vi "Needle Valve labVIEW Code-Original.vi"() -> ()   [LabVIEW 2025]
uses:
  e7797c04-791b-4eea-89a1-5a3bec2431d3.vi
  bf5fd3a0-ddf8-478e-bb95-a39885d33854.vi
  0285ecf2-4d18-4427-ace1-61b1951a0741.vi
  843b8d60-a9e3-46f8-8afe-ca8ffa5d81a2.vi
  fe75afdf-d463-4dd5-8739-de0ca1ff0544.vi
  <vilib>/gmath/NI_Gmath.lvlib
  d3b0afdc-d7ac-4f1a-8ecc-0aeb21fe1e80.vi
  c8945bc9-af31-4a2e-9b52-27840c61c0f1.vi
  <vilib>/Utility/file.llb/Write Delimited Spreadsheet (DBL).vi
  <vilib>/Utility/file.llb/Read Delimited Spreadsheet (DBL).vi
  <vilib>/addons/_office/excel.llb/Excel Easy Table (num).vi
  <vilib>/Utility/NIReport.llb/NI_report.lvclass
  <vilib>/Utility/NIReport.llb/Report Type.ctl
  <vilib>/Utility/NIReport.llb/NI_ReportGenerationCore.lvlib
  0d300616-a92e-4ad7-b5ed-aabe3c94486a.vi
  <vilib>/Instr/_visa.llb/VISA Configure Serial Port (Instr).vi
  <vilib>/addons/_office/excel.llb/Excel Easy Table (str).vi
panel:
  in  "Sensor Values Excel Sheet Name":string
  in  "?":u32(colorbox)
  out "Waveform Chart":dbl[](graph)
  in  "Loop Iteration":i32
  in  "Saved Sensor Values":path
  in  "Mach 2.1 Table Excel Sheet Name":string
  in  "Mach 3.0 Table Excel Sheet Name":string
  out "Mach # duration (s)":dbl
  in  "Mach Tables Location":path
  out "Output Mach #\n(For Reference Only)":dbl format="%#_4g"
  out "Motor Signal":string
  out "?":dbl format="%.4f"
  out "Output Mach #\n(For Reference Only)":dbl format="%#_4g"
  out "Motor Signal":string
  out "?":dbl format="%.3f"
  in  "Seclect Spike":enum16{"Mach 2.1 Spike", "Mach 3.0 Spike"}(ring)
  in  "?":dbl
  out "Motor Signal":string
  in  "?":dbl[][](array[numeric])=[[10.0, 10.0, 0.0, 22.0]]
  in  "stop program":bool
  in  "?":bool
  out "?":dbl format="%.4f"
  in  "Select Mach Number":dbl[](array[numeric])
  out "Spike Position":dbl[][](graph)
  out "Arduino Error":errorcluster
  in  "VISA resource Port":refnum<visa-resource-name>
  out "?":dbl format="%.3f"
  out "?":dbl format="%.3f"
  in  "Set Spike Position (in)":dbl(slide) scale=0.0..0.5
  in  "Mach Number, Spike Distance (in) (3.0M)":dbl[][](array[numeric])=[[10.0, 10.0, 0.0, 22.0]]
  in  "Mach Number, Spike Distance (in) (2.1M)":dbl[][](array[numeric])=[[10.0, 10.0, 0.0, 22.0]]
  out "?":dbl(slide) scale=0.0..1000.0
  out "Stagnation Flow Temp (K)\n(For Refrence only)":dbl
  out "Stagnation pressure (PSIA)\n(For Refrence only)":dbl
  in  "Sensor Offsets":dbl[](array[numeric])=[10.0, 10.0, 0.0, 22.0]
  in  "Sensor K-values":dbl[](array[numeric])=[10.0, 10.0, 0.0, 22.0]
  in  "?":bool
  in  "?":bool
  in  "?":bool
  out "Screw RPM (95% efficency assumed)":dbl
  out "Spike Linear Speed (in/s)\n(For Reference Only)":dbl format="%#_4g"
  in  "Motor Control Loop Rate (ms)":dbl
  out "Set Motor RPM":dbl(knob) scale=0.0..200.0
  in  "Flight Profile Mode":bool
  in  "Set Mach # Mode":bool
  in  "Manual Positioning Mode":bool
  in  "Stop Sensors":bool
  in  "Sensor Loop Rate (ms)":dbl
  out "Time Since Start (s)\n(For Reference Only)":dbl format="%.2f"
  in  "loop stop 2":bool
  in  "loop stop 1":bool
  in  "Sensor Inputs Location":path
  in  "Start Sensors":bool
  in  "Load Inputs":bool
  in  "Save Inputs":bool
  out "Potentiometer distance\n(For Reference Only)":dbl
  out "Port":i32
  out "ConnectionType":i32
  out "DeviceType":i32
  out "Labjack error":errorcluster
  # "34HS59-6004S Motor Torque Curve (For Reference)"
  # "Labjack/Arduino Resources"
  # "Inputs and LabJack Sensor Monitors"
  # "Mach Number Tables"
  # "Mach 3.0 Spike Table"
  # "Mach 2.1 Spike Table"
  # "Motor RPM >200 RPM"
  # "Potentiometer"
  # "Inefficent Torque for High Mass Flow/Thrust Tests"
  # "Ducer"
  # "Thermocouple"
  # "Motor RPM < 200 RPM"
  # "(Labjack Auto-Populates)"
  # "(dial indicator for range reference)"
  # "COM Port for Arduino"
  # "Stop sensors automatically saves sensor data"
  # "Distance to Go (in)\n(For Reference Only)"
  # "Output Mach #\n(For Reference Only)"
  # "Column one: selected Mach numbers"
  # "Profile Control Array"
  # "Column Two: selected timing for each Mach number (seconds)"
  # "Distance to Go (in)\n(For Reference Only)"
  # "Profile will be completed at first Mach number = \"0\""
  # "Distance to Go (in)\n(For Reference Only)"
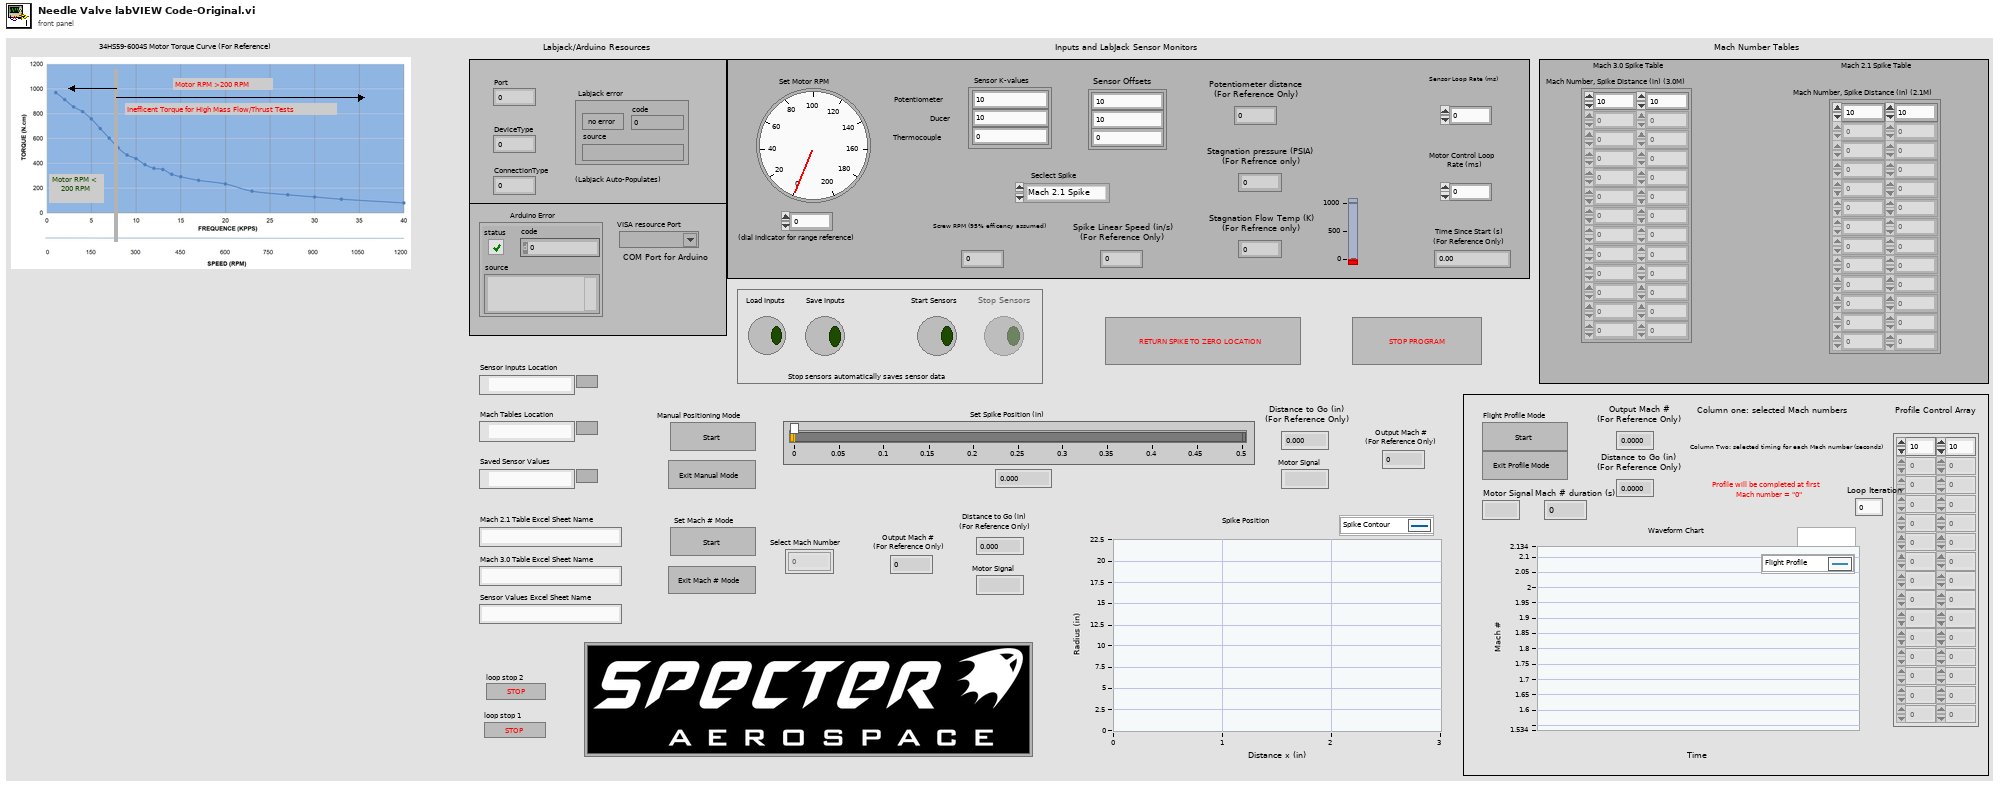
[diagram p1: front panel]
types:
  T1 = enum16{"Save Data", "Idle Mode", "Manual Positioning Mode", "Set Mach # mode", "Flight Profile Mode"}
  T2 = enum16{"save data", "Start sensors", "save values", "load Values", "Idle"}
  T3 = enum8{"Enabled", "Disabled", "Disabled and Grayed Out"}
  T4 = typedef "NI_ReportGenerationCore.lvlib/Report Type.ctl" = enum16{"HTML", "Word", "Excel"}
  T5 = enum16{"Left Button", "Center Button", "Right Button", "Window Close"}
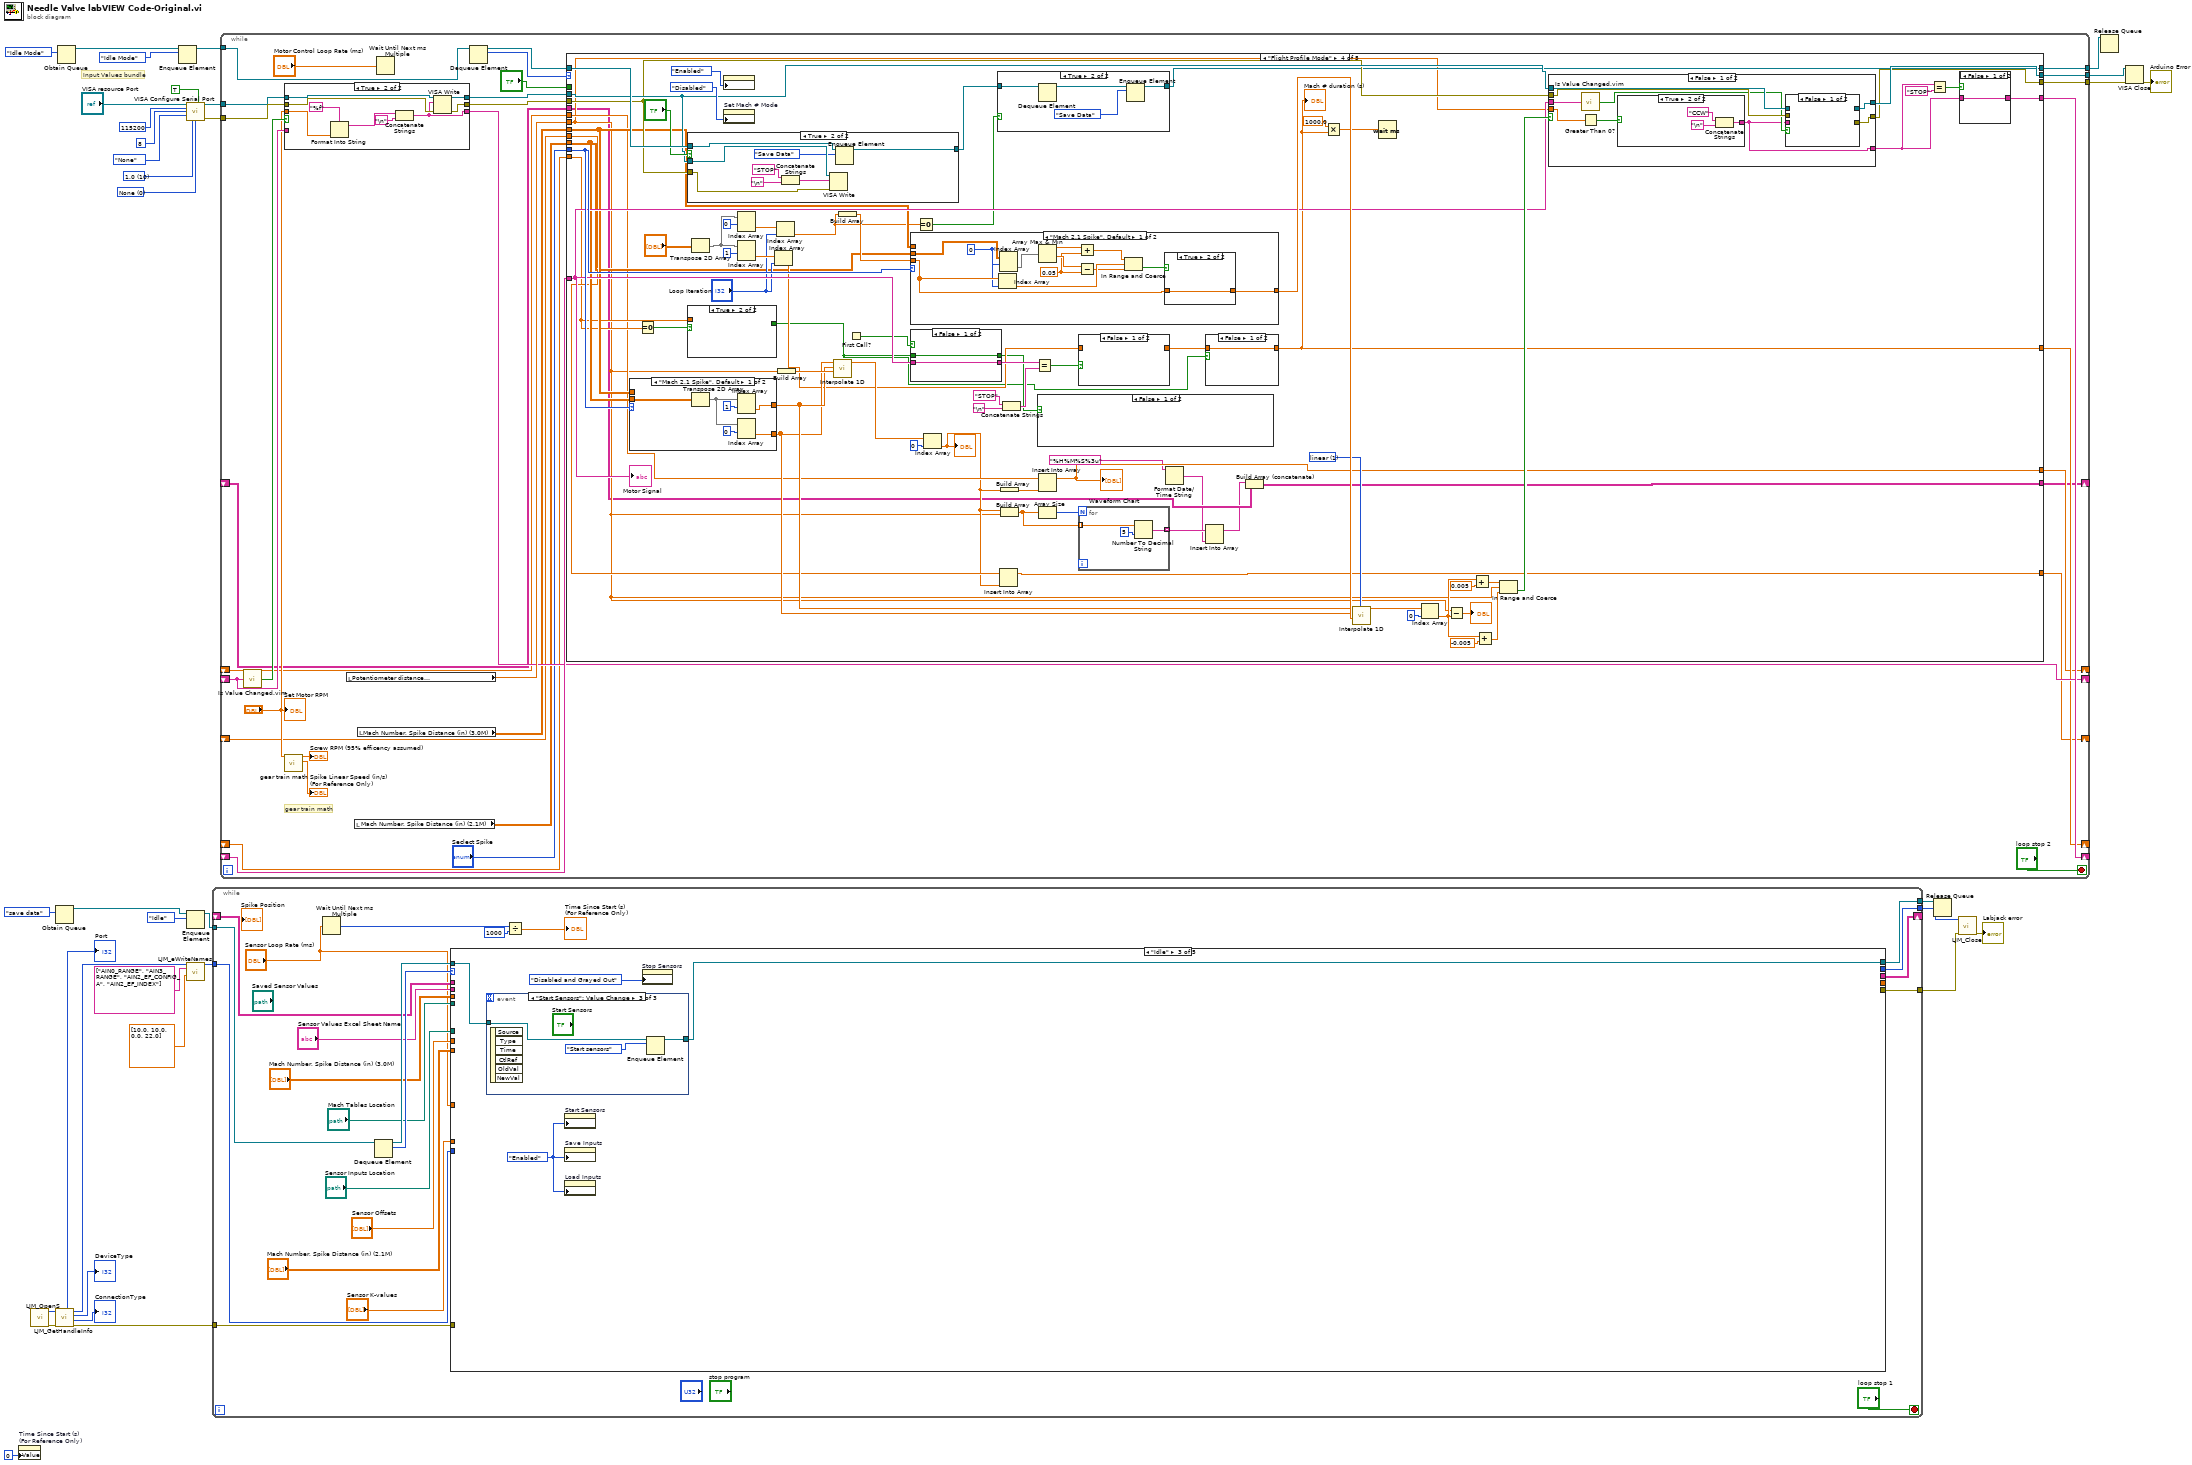
[diagram p0: block diagram]
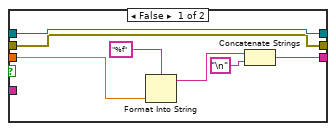
[diagram p2: hidden frame]
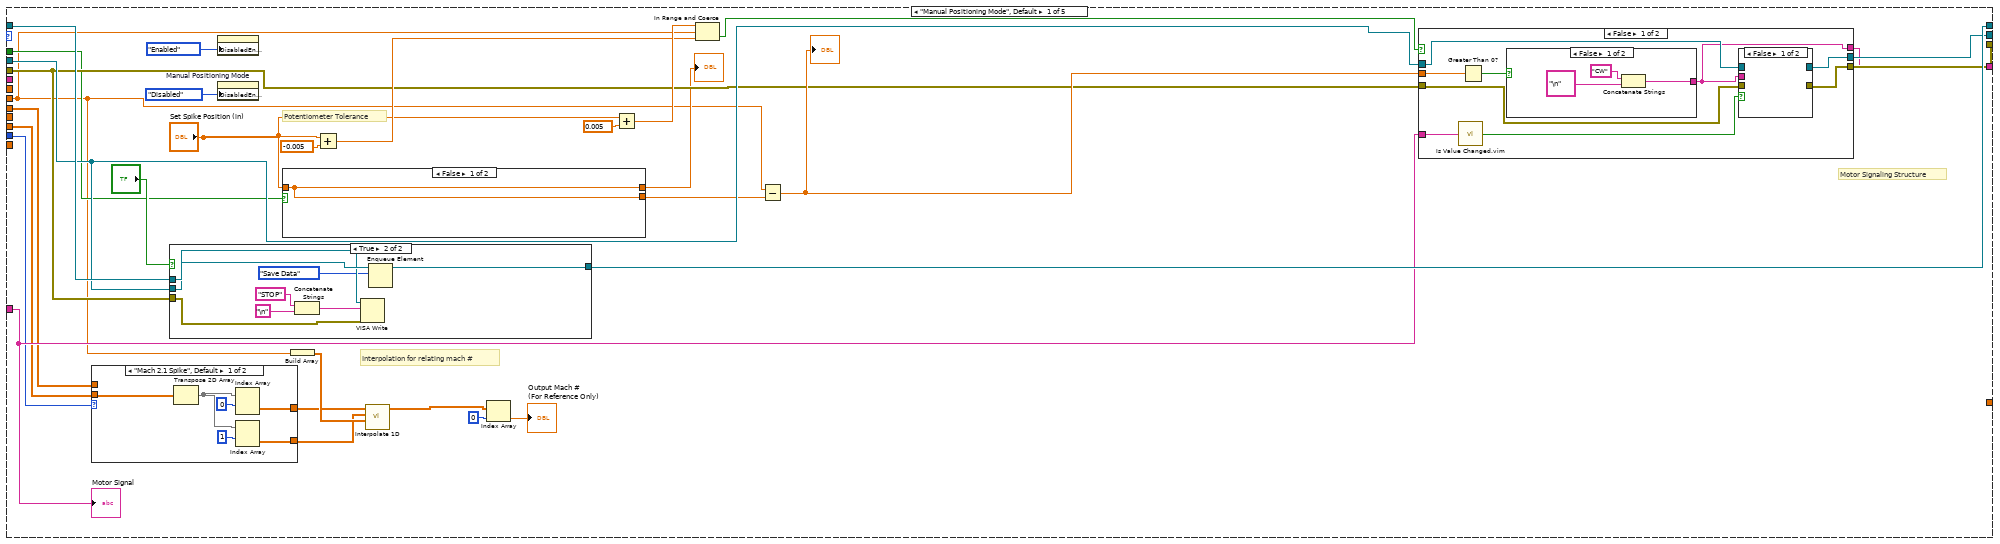
[diagram p3: hidden frame]
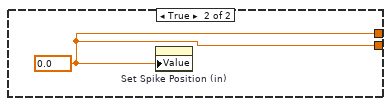
[diagram p4: hidden frame]
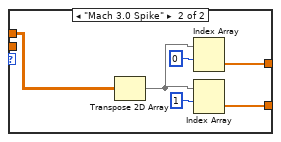
[diagram p5: hidden frame]
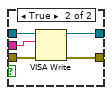
[diagram p6: hidden frame]
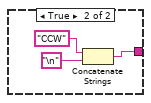
[diagram p7: hidden frame]
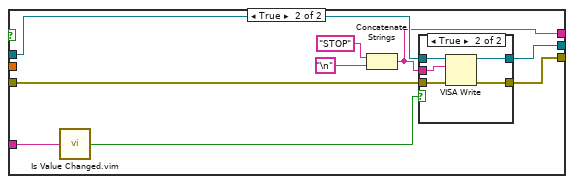
[diagram p8: hidden frame]
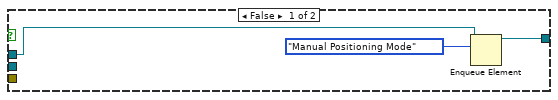
[diagram p10: hidden frame]
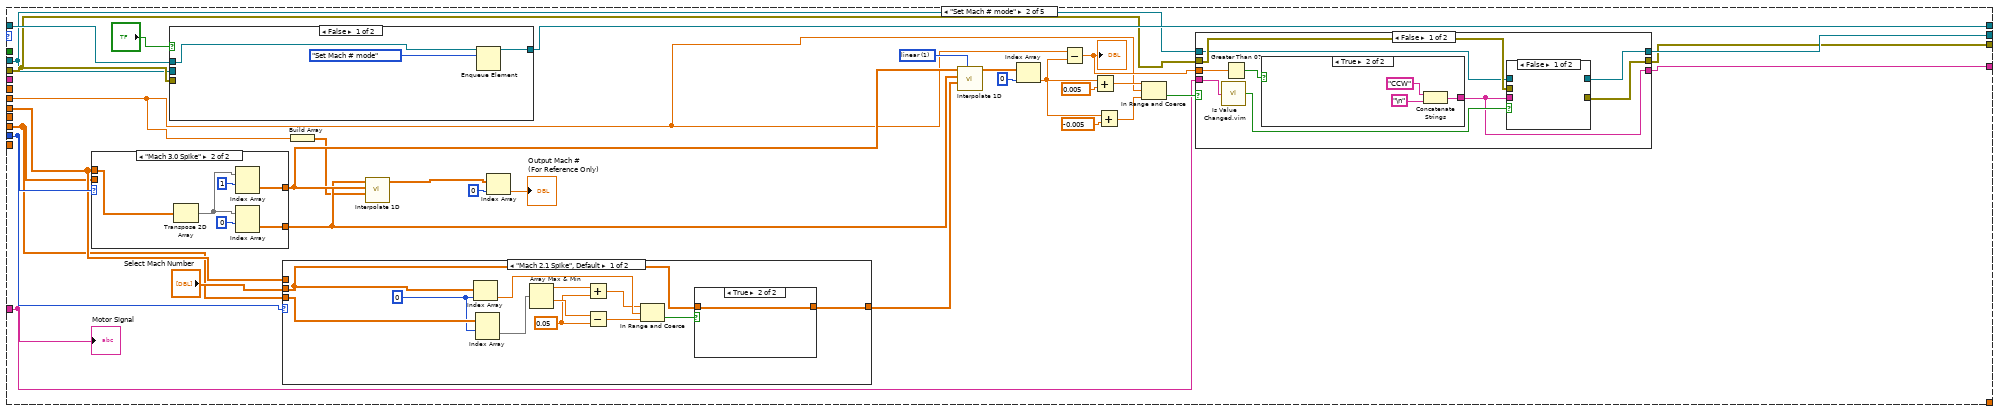
[diagram p11: hidden frame]
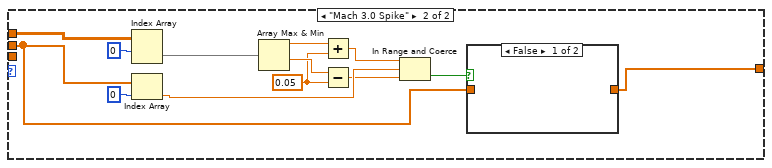
[diagram p13: hidden frame]
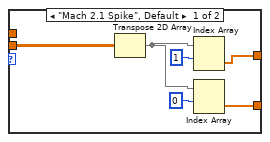
[diagram p15: hidden frame]
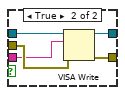
[diagram p16: hidden frame]
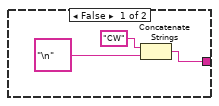
[diagram p17: hidden frame]
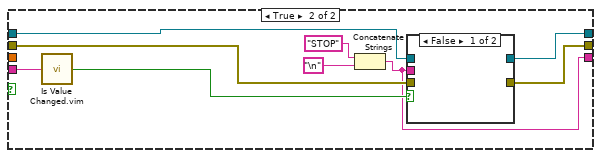
[diagram p18: hidden frame]
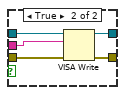
[diagram p19: hidden frame]
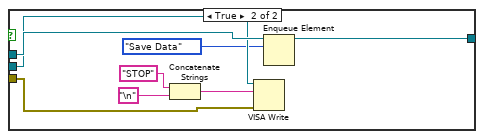
[diagram p20: hidden frame]
diagram:
  w5 = u16 0 items=["None", "XON/XOFF", "RTS/CTS", "XON/XOFF & RTS/CTS", "DTR/DSR", "XON/XOFF & DTR/DSR"] ("flow control (0:none)")
  w6 = u16 10 items=["1.0"=10, "1.5"=15, "2.0"=20] ("stop bits (10: 1 bit)")
  # "Input Values bundle"
  n1 = property on="Time Since Start (s)\n(For Reference Only)" class="DigNum (strict)"("Value"=u32 0 ("Time Since Start (s)\n(For Reference Only) 2")) -> ()  [unwired: 2 in, 2 out]
  n2 = call "LJM_OpenS.vi"() -> ("error out"=w31:errorcluster, "Handle"=w35:i32)  [unwired: 10 in]
  n3 = Obtain Queue(element data type=T2."save data" ("Enum")) -> (queue out=w24:refnum<queue>)  [unwired: 4 in, 2 out]
  n4 = call "LJM_GetHandleInfo.vi"("error in"=w31, "Handle In"=w35) -> ("error out"=w30:errorcluster, "ConnectionType"=→"ConnectionType":i32, "DeviceType"=→"DeviceType":i32, "Handle Out"=w17:i32, "Port"=→"Port":i32)  [unwired: 2 in, 3 out]
  n5 = Obtain Queue(element data type=T1."Idle Mode") -> (queue out=w26:refnum<queue>)  [unwired: 4 in, 2 out]
  n6 = Enqueue Element(queue=w26, element=T1."Idle Mode") -> (queue out=w25:refnum<queue>)  [unwired: 2 in, 2 out]
  n7 = call-poly "VISA Configure Serial Port"("VISA resource name"="VISA resource Port", "Enable Termination\nChar (T)"=TRUE ("Enable Termination\nChar (T)"), "baud rate (9600)"=u32 115200, "data bits (8)"=u16 8, "parity (0:none)"=enum16{"None", "Odd", "Even", "Mark", "Space"}."None", "stop bits (10: 1 bit)"=w6, "flow control (0:none)"=w5) -> ("VISA resource name out"=w3:refnum<visa-resource-name>, "error out"=w4:errorcluster)  [unwired: 7 in]
  n8 = Enqueue Element(queue=w24, element=T2."Idle" ("Enum")) -> (queue out=w23:refnum<queue>)  [unwired: 2 in, 2 out]
  n9 = call "LJM_eWriteNames.vi"("Handle In"=w17, "aNames"=string[] ["AIN0_RANGE", "AIN3_RANGE", "AIN2_EF_CONFIG_A", "AIN2_EF_INDEX"], "aValuesIn"=dbl[] [10.0, 10.0, 0.0, 22.0]) -> ("Handle Out"=w16:i32)  [unwired: 10 in, 2 out]
  n10 = while {
    tunnel: w30 -> [w58]
    tunnel: [w57] -> w29
    tunnel: w16 -> [w56]
    tunnel: [w55] -> w28
    tunnel: w23 -> [w54]
    tunnel: [w51] -> w21
    shift-right: [w40] -> _
    shift-left: _ -> [w39]
    stop <- "loop stop 1" stop-if-true
    n11 = Wait Until Next ms Multiple(millisecond multiple="Sensor Loop Rate (ms)") -> (millisecond timer value=w49:u32)
    n12 = Dequeue Element(queue=w54) -> (queue out=w52:refnum<queue>, element=w53:T2)  [unwired: 2 in, 2 out]
    n13 = case shown="\"Idle\"" w53 {
      tunnel: w58 -> [_ _ _ w180 _]
      tunnel: [_ _ _ w179 _] -> w57
      tunnel: w56 -> [_ _ _ w182 _]
      tunnel: [_ _ _ w181 _] -> w55
      tunnel: w52 -> [w80 w115 w150 w187 w211]
      tunnel: [w79 w114 w149 w186 w209] -> w51
      tunnel: [_ _ _ w171 _] -> _
      tunnel: "Sensor Offsets" -> [w76 _ _ w176 _]
      tunnel: "Sensor K-values" -> [w75 _ _ w175 _]
      tunnel: "Sensor Inputs Location" -> [w72 w112 _ _ _]
      tunnel: "Mach Tables Location" -> [w69 w111 _ _ _]
      tunnel: "Mach Number, Spike Distance (in) (2.1M)" -> [w68 _ _ _ _]
      tunnel: "Mach Number, Spike Distance (in) (3.0M)" -> [w70 _ _ _ _]
      tunnel: [_ _ _ w163 _] -> w40
      tunnel: w39 -> [_ _ _ w162 w204]
      tunnel: "Sensor Values Excel Sheet Name" -> [_ _ _ _ w202]
      tunnel: "Sensor Loop Rate (ms)" -> [w60 _ _ _ _]
      frame "save values", Default {
        w63 = string[] ["Mach #", "Spike Distance (in)"] ("column headers")
        w74 = Report_Type."Excel" ("report type")
        n14 = local read "Motor Control Loop Rate (ms)"() -> (w62:dbl)
        n15 = Enqueue Element(queue=w80, element=T2."Idle" ("Enum")) -> (queue out=w79:refnum<queue>)  [unwired: 2 in, 2 out]
        n16 = local read "Set Motor RPM"() -> (w73:dbl)
        n17 = Build Array(w60) -> (w59:dbl[])
        n18 = Build Array(w62) -> (w61:dbl[])
        n19 = Build Array(w73) -> (w77:dbl[])
        n20 = Build Array(w75, w76, w77, w59, w61) -> (w71:dbl[][])
        n21 = flat-sequence {
          tunnel: w72 -> [w84]
          tunnel: w71 -> [w83]
          tunnel: w69 -> [w93]
          tunnel: w70 -> [w92]
          tunnel: w65 -> [w89]
          tunnel: "Mach 3.0 Table Excel Sheet Name" -> [w88]
          tunnel: w63 -> [w87]
          tunnel: w69 -> [w105]
          tunnel: w68 -> [w104]
          tunnel: w67 -> [w101]
          tunnel: "Mach 2.1 Table Excel Sheet Name" -> [w100]
          tunnel: w63 -> [w99]
          frame #0 {
            n22 = Two Button Dialog(message="Save Sensor Values/Inputs?" ("Message")) -> (T button?=w82:bool)  [unwired: 2 in]
            n23 = case shown="True" w82 {
              tunnel: w84 -> [_ w86]
              tunnel: w83 -> [_ w85]
              frame False {
              }
              frame True {
                n24 = call-poly <vilib>:"Write Delimited Spreadsheet.vi"("file path (dialog if empty)"=w86, "2D data"=w85) -> ()  [unwired: 12 in, 2 out]
              }
            }
          }
          frame #1 {
            n25 = Two Button Dialog(message="Save Mach 3.0 Table" ("Message")) -> (T button?=w90:bool)  [unwired: 2 in]
            n26 = case shown="True" w90 {
              tunnel: w93 -> [_ w98]
              tunnel: w92 -> [_ w96]
              tunnel: w89 -> [_ w97]
              tunnel: w88 -> [_ w95]
              tunnel: w87 -> [_ w94]
              frame False {
              }
              frame True {
                n27 = call-poly <vilib>:"Write Delimited Spreadsheet.vi"("file path (dialog if empty)"=w98, "2D data"=w96) -> ()  [unwired: 12 in, 2 out]
                n28 = call-poly <vilib>:"Excel Easy Table.vi"("report in"=w97, "text data"=w96, "name (\"\")"=w95, "column headers"=w94) -> ()  [unwired: 7 in, 5 out]
              }
            }
          }
          frame #2 {
            n29 = Two Button Dialog(message="Save Mach 2.1 Table" ("Message")) -> (T button?=w102:bool)  [unwired: 2 in]
            n30 = case shown="True" w102 {
              tunnel: w105 -> [_ w110]
              tunnel: w104 -> [_ w108]
              tunnel: w101 -> [_ w109]
              tunnel: w100 -> [_ w107]
              tunnel: w99 -> [_ w106]
              frame False {
              }
              frame True {
                n31 = call-poly <vilib>:"Excel Easy Table.vi"("report in"=w109, "text data"=w108, "name (\"\")"=w107, "column headers"=w106) -> ()  [unwired: 7 in, 5 out]
                n32 = call-poly <vilib>:"Write Delimited Spreadsheet.vi"("file path (dialog if empty)"=w110, "2D data"=w108) -> ()  [unwired: 12 in, 2 out]
              }
            }
          }
        }
        n33 = call <vilib>:"Create Report.vi"("Report Type"=w74) -> ("report out"=w65:refnum<class "NI_report.lvclass">)  [unwired: 13 in, 1 out]
        n34 = call <vilib>:"Create Report.vi"("Report Type"=w74) -> ("report out"=w67:refnum<class "NI_report.lvclass">)  [unwired: 13 in, 1 out]
      }
      frame "load Values" {
        n35 = flat-sequence {
          tunnel: w112 -> [w118]
          tunnel: w111 -> [w139]
          tunnel: w111 -> [w144]
          frame #0 {
            n36 = Two Button Dialog(message="Sensor and RPM File Selection" ("Message")) -> (T button?=w116:bool)  [unwired: 2 in]
            n37 = case shown="True" w116 {
              tunnel: w118 -> [_ w128]
              frame False {
              }
              frame True {
                # "Loading Motor RPM"
                n38 = call-poly <vilib>:"Read Delimited Spreadsheet.vi"("file path (dialog if empty)"=w128) -> ("all rows"=w120:dbl[][])  [unwired: 9 in, 5 out]
                n39 = Index Array(array=w120, index (row)=0) -> (element=w135:dbl[])  [unwired: 1 in]
                n40 = Index Array(array=w120, index (row)=2) -> (element=w131:dbl[])  [unwired: 1 in]
                n41 = Index Array(array=w120, index (row)=1) -> (element=w133:dbl[])  [unwired: 1 in]
                n42 = property on="Sensor K-values" class="Arr (strict)"("Value"=w135) -> ()  [unwired: 2 in, 2 out]
                n43 = property on="Sensor Offsets" class="Arr (strict)"("Value"=w133) -> ()  [unwired: 2 in, 2 out]
                n44 = Index Array(array=w120, index (row)=3) -> (element=w126:dbl[])  [unwired: 1 in]
                n45 = Index Array(array=w120, index (row)=4) -> (element=w122:dbl[])  [unwired: 1 in]
                n46 = Index Array(array=w131, index=0) -> (element=w129:dbl)
                n47 = property class="DigNum (strict)"("Value"=w129) -> ()  [unwired: 2 in, 2 out]
                n48 = Index Array(array=w126, index=0) -> (element=w124:dbl)
                n49 = Index Array(array=w122, index=0) -> (element=w119:dbl)
                n50 = property on="Motor Control Loop Rate (ms)" class="DigNum (strict)"("Value"=w119) -> ()  [unwired: 2 in, 2 out]
                n51 = property on="Sensor Loop Rate (ms)" class="DigNum (strict)"("Value"=w124) -> ()  [unwired: 2 in, 2 out]
              }
            }
          }
          frame #1 {
            n52 = Two Button Dialog(message="Mach 2.1 Table Selection" ("Message")) -> (T button?=w137:bool)  [unwired: 2 in]
            n53 = case shown="True" w137 {
              tunnel: w139 -> [_ w140]
              frame False {
              }
              frame True {
                n54 = call-poly <vilib>:"Read Delimited Spreadsheet.vi"("file path (dialog if empty)"=w140) -> ("all rows"=w141:dbl[][])  [unwired: 9 in, 5 out]
                n55 = property on="Mach Number, Spike Distance (in) (2.1M)" class="Arr (strict)"("Value"=w141) -> ()  [unwired: 2 in, 2 out]
              }
            }
          }
          frame #2 {
            n56 = Two Button Dialog(message="Mach 3.0 Table Selection" ("Message")) -> (T button?=w142:bool)  [unwired: 2 in]
            n57 = case shown="True" w142 {
              tunnel: w144 -> [_ w146]
              frame False {
              }
              frame True {
                n58 = call-poly <vilib>:"Read Delimited Spreadsheet.vi"("file path (dialog if empty)"=w146) -> ("all rows"=w145:dbl[][])  [unwired: 9 in, 5 out]
                n59 = property on="Mach Number, Spike Distance (in) (3.0M)" class="Arr (strict)"("Value"=w145) -> ()  [unwired: 2 in, 2 out]
              }
            }
          }
        }
        n60 = Enqueue Element(queue=w115, element=T2."Idle" ("Enum")) -> (queue out=w114:refnum<queue>)  [unwired: 2 in, 2 out]
      }
      frame "Idle" {
        w148 = T3."Enabled" ("Disabled")
        n61 = event shown="[2] \"Start Sensors\": Value Change" {
          selector: _ -> [_ _ _]
          dyn-events: _ -> [_ _ _]
          timeout: _ -> [_ _ _]
          tunnel: w150 -> [w153 w156 w159]
          tunnel: [w152 w155 w158] -> w149
          event "Save Inputs": Value Change {
            n62 = event-data() -> ()  [unwired: 1 in, 6 out]
            n63 = Enqueue Element(queue=w153, element=T2."save values" ("Enum")) -> (queue out=w152:refnum<queue>)  [unwired: 2 in, 2 out]
          }
          event "Load Inputs": Value Change {
            n64 = event-data() -> ()  [unwired: 1 in, 6 out]
            n65 = Enqueue Element(queue=w156, element=T2."load Values" ("Enum")) -> (queue out=w155:refnum<queue>)  [unwired: 2 in, 2 out]
          }
          event "Start Sensors": Value Change {
            n66 = event-data() -> ()  [unwired: 1 in, 6 out]
            n67 = Enqueue Element(queue=w159, element=T2."Start sensors" ("Enum")) -> (queue out=w158:refnum<queue>)  [unwired: 2 in, 2 out]
          }
        }
        n68 = property on="Start Sensors" class="Bool"("DisabledEnum"=w148) -> ()  [unwired: 2 in, 2 out]
        n69 = property on="Save Inputs" class="Bool"("DisabledEnum"=w148) -> ()  [unwired: 2 in, 2 out]
        n70 = property on="Load Inputs" class="Bool"("DisabledEnum"=w148) -> ()  [unwired: 2 in, 2 out]
        n71 = property on="Stop Sensors" class="Bool"("DisabledEnum"=T3."Disabled and Grayed Out" ("Disabled")) -> ()  [unwired: 2 in, 2 out]
      }
      frame "Start sensors" {
        (unwired) 5 ("sample length")
        w184 = T3."Disabled and Grayed Out" ("Disabled")
        # "Sensor Calibration and LabJack Read"
        n72 = Array Size(array=w176) -> (size(s)=w177:i32)
        n73 = property on="Stop Sensors" class="Bool"("DisabledEnum"=T3."Enabled" ("Disabled")) -> ()  [unwired: 2 in, 2 out]
        n74 = call "LJM_eReadNames.vi"("Handle In"=w182, "aNames"=string[] ["AIN0", "AIN3", "AIN2_EF_READ_A"], "error in"=w180) -> ("Handle Out"=w181:i32, "aValuesOut"=w168:dbl[], "error out"=w179:errorcluster)  [unwired: 9 in, 1 out]
        n75 = property on="Save Inputs" class="Bool"("DisabledEnum"=w184) -> ()  [unwired: 2 in, 2 out]
        n76 = property on="Start Sensors" class="Bool"("DisabledEnum"=w184) -> ()  [unwired: 2 in, 2 out]
        n77 = property on="Load Inputs" class="Bool"("DisabledEnum"=w184) -> ()  [unwired: 2 in, 2 out]
        n78 = for {
          N: w177 -> [_]
          tunnel: w176 -> [w192] mode=indexing
          tunnel: w175 -> [w193] mode=indexing
          tunnel: w168 -> [w195] mode=indexing
          tunnel: [w191] -> w166 mode=indexing
          n79 = Multiply(x=w193, y=w195) -> (x*y=w194:dbl)
          n80 = Add(x=w192, y=w194) -> (x+y=w191:dbl)
        }
        n81 = case shown="True" "Stop Sensors" {
          tunnel: w187 -> [w198 w201]
          tunnel: [w197 w200] -> w186
          frame False {
            n82 = Enqueue Element(queue=w198, element=T2."Start sensors" ("Enum")) -> (queue out=w197:refnum<queue>)  [unwired: 2 in, 2 out]
          }
          frame True {
            n83 = Enqueue Element(queue=w201, element=T2."save data") -> (queue out=w200:refnum<queue>)  [unwired: 2 in, 2 out]
          }
        }
        n84 = Array Size(array=w166) -> (size(s)=w167:i32)
        n85 = Index Array(array=w166, index=enum16{"Potentiometer", "Ducer", "Thermocouple"}."Potentiometer" ("Enum")) -> (element=w171:dbl)
        "Potentiometer distance\n(For Reference Only)" <- w171
        n86 = Index Array(array=w166, index=enum16{"Potentiometer", "Ducer", "Thermocouple"}."Thermocouple" ("Enum")) -> (element=→"?" →"Stagnation Flow Temp (K)\n(For Refrence only)":dbl)
        n87 = for {
          N: w167 -> [_]
          tunnel: w166 -> [w190] mode=indexing
          tunnel: [w188] -> w165 mode=indexing
          n88 = Number To Decimal String(number=w190, width (-)=i16 5) -> (decimal integer string=w188:string)
        }
        n89 = Index Array(array=w166, index=enum16{"Potentiometer", "Ducer", "Thermocouple"}."Ducer" ("Enum")) -> (element=→"Stagnation pressure (PSIA)\n(For Refrence only)":dbl)
        n90 = Format Date/Time String(time format string (%c)="%H%M%S%3u") -> (date/time string=w160:string)  [unwired: 2 in]
        n91 = Insert Into Array(array=w165, new element=w160) -> (w164:string[])  [unwired: 1 in]
        n92 = Build Array (concatenate)(w164, w162) -> (w163:string[][])
      }
      frame "save data" {
        n93 = Enqueue Element(queue=w211, element=T2."Idle") -> (queue out=w209:refnum<queue>)  [unwired: 2 in, 2 out]
        n94 = Two Button Dialog(message="Save sensor Values?" ("Message")) -> (T button?=w207:bool)  [unwired: 2 in]
        n95 = call <vilib>:"Create Report.vi"("Report Type"=Report_Type."Excel" ("report type")) -> ("report out"=w206:refnum<class "NI_report.lvclass">)  [unwired: 13 in, 1 out]
        n96 = case shown="True" w207 {
          tunnel: w206 -> [_ w213]
          tunnel: string[] ["Spike position (in)", "Flow Pressure (PSIA)", "Flow Temperature (K)", "Time (s)"] ("column headers") -> [_ w215]
          tunnel: w204 -> [_ w214]
          tunnel: w202 -> [_ w212]
          frame False {
          }
          frame True {
            n97 = call-poly <vilib>:"Excel Easy Table.vi"("report in"=w213, "text data"=w214, "name (\"\")"=w212, "column headers"=w215) -> ()  [unwired: 7 in, 5 out]
          }
        }
      }
    }
    n98 = Divide(x=w49, y=u32 1000) -> (x/y=→"Time Since Start (s)\n(For Reference Only)":dbl)
  }
  n99 = while {
    tunnel: w25 -> [w248]
    tunnel: [w246] -> w20
    tunnel: [w241] -> w11
    tunnel: [w240] -> w10
    shift-right: [w239] -> _
    shift-left: _ -> [w238]
    tunnel: w4 -> [w237]
    tunnel: w3 -> [w236]
    shift-right: [w232] -> _
    shift-left: _ -> [w231]
    shift-right: [w223] -> _
    shift-left: _ -> [w222]
    shift-right: [w221] -> _
    shift-left: _ -> [w220]
    shift-right: [w219] -> _
    shift-left: _ -> [w218]
    shift-right: [w217] -> _
    shift-left: _ -> [w216]
    stop <- "loop stop 2" stop-if-true
    # "gear train math"
    n100 = call "Is Value Changed.vim"("value"=w231) -> ("changed or first call?"=w233:bool)
    n101 = case shown="True" w233 {
      tunnel: w237 -> [w254 w264]
      tunnel: [w250 w256] -> w232
      tunnel: w236 -> [w255 w263]
      tunnel: [w254 w262] -> w235
      tunnel: [w255 w259] -> w234
      tunnel: "?" -> [w253 w261]
      tunnel: w231 -> [_ _]
      frame False {
        n102 = Format Into String(format string="%f", w253) -> (resulting string=w251:string)  [unwired: 2 in, 1 out]
        n103 = Concatenate Strings(w251, "\n" ("string")) -> (w250:string)
      }
      frame True {
        n104 = Format Into String(format string="%f", w261) -> (resulting string=w258:string)  [unwired: 2 in, 1 out]
        n105 = Concatenate Strings(w258, "\n" ("string")) -> (w256:string)
        n106 = VISA Write(VISA resource name=w263, write buffer=w256, error in (no error)=w264) -> (VISA resource name out=w259:refnum<visa-resource-name>, error out=w262:errorcluster)  [unwired: 1 out]
      }
    }
    n107 = call "gear train math.vi"("Numeric in"="?") -> ("Numeric 3"=→"Spike Linear Speed (in/s)\n(For Reference Only)":dbl, "Numeric out"=→"Screw RPM (95% efficency assumed)":dbl)  [unwired: 9 in]
    n108 = local read "Potentiometer distance\n(For Reference Only)"() -> (w242:dbl)
    n109 = local read "Mach Number, Spike Distance (in) (2.1M)"() -> (w225:dbl[][])
    n110 = local read "Mach Number, Spike Distance (in) (3.0M)"() -> (w224:dbl[][])
    n111 = Wait Until Next ms Multiple(millisecond multiple="Motor Control Loop Rate (ms)") -> ()  [unwired: 1 out]
    n112 = Dequeue Element(queue=w248) -> (queue out=w245:refnum<queue>, element=w247:T1)  [unwired: 2 in, 2 out]
    n113 = case shown="\"Flight Profile Mode\"" w247 {
      tunnel: [w294 w379 w480 w514 w677] -> w246
      tunnel: w245 -> [w295 w378 w481 w564 w679]
      tunnel: w242 -> [w265 w358 _ w499 _]
      tunnel: w234 -> [w282 w376 w472 w546 _]
      tunnel: [w286 w375 w472 w549 _] -> w241
      tunnel: w235 -> [w281 w377 w471 w545 _]
      tunnel: [w285 w374 w471 w548 _] -> w240
      tunnel: [w284 w373 _ w542 _] -> w239
      tunnel: w238 -> [w283 w372 _ w538 _]
      tunnel: "Seclect Spike" -> [w278 w369 _ w550 _]
      tunnel: w225 -> [w277 w355 _ w517 _]
      tunnel: w224 -> [w276 w356 _ w518 _]
      tunnel: "?" -> [w269 _ _ _ _]
      tunnel: [_ _ _ w510 _] -> w223
      tunnel: w222 -> [_ _ _ w505 _]
      tunnel: [_ _ _ w506 _] -> w221
      tunnel: w220 -> [_ _ _ w507 _]
      tunnel: [_ _ _ w502 _] -> w219
      tunnel: w218 -> [_ _ _ w501 _]
      tunnel: [_ _ _ w497 _] -> w217
      tunnel: w216 -> [_ _ _ w496 w673]
      frame "Manual Positioning Mode", Default {
        # "Motor Signaling Structure"
        # "Potentiometer Tolerance"
        # "Interpolation for relating mach #"
        n114 = case shown="\"Mach 2.1 Spike\", Default" w278 {
          tunnel: w277 -> [w301 _]
          tunnel: [w303 w308] -> w274
          tunnel: [w302 w309] -> w273
          tunnel: w276 -> [_ w305]
          frame "Mach 2.1 Spike", Default {
            n115 = Transpose 2D Array(2D array=w301) -> (transposed array=w300:dbl[][])
            n116 = Index Array(array=w300, index (row)=0) -> (element=w302:dbl[])  [unwired: 1 in]
            n117 = Index Array(array=w300, index (row)=1) -> (element=w303:dbl[])  [unwired: 1 in]
          }
          frame "Mach 3.0 Spike" {
            n118 = Transpose 2D Array(2D array=w305) -> (transposed array=w304:dbl[][])
            n119 = Index Array(array=w304, index (row)=0) -> (element=w309:dbl[])  [unwired: 1 in]
            n120 = Index Array(array=w304, index (row)=1) -> (element=w308:dbl[])  [unwired: 1 in]
          }
        }
        n121 = case shown="True" "?" {
          tunnel: w295 -> [w346 w354]
          tunnel: [w345 w353] -> w294
          tunnel: w282 -> [_ w349]
          tunnel: w281 -> [_ w348]
          frame False {
            n122 = Enqueue Element(queue=w346, element=T1."Manual Positioning Mode") -> (queue out=w345:refnum<queue>)  [unwired: 2 in, 2 out]
          }
          frame True {
            n123 = Concatenate Strings("STOP" ("write buffer"), "\n" ("write buffer")) -> (w352:string)
            n124 = VISA Write(VISA resource name=w349, write buffer=w352, error in (no error)=w348) -> ()  [unwired: 3 out]
            n125 = Enqueue Element(queue=w354, element=T1."Save Data") -> (queue out=w353:refnum<queue>)  [unwired: 2 in, 2 out]
          }
        }
        n126 = property class="Bool"("DisabledEnum"=T3."Enabled" ("Disabled")) -> ()  [unwired: 2 in, 2 out]
        n127 = property on="Manual Positioning Mode" class="Bool"("DisabledEnum"=T3."Disabled" ("Disabled")) -> ()  [unwired: 2 in, 2 out]
        n128 = case shown="False" w269 {
          tunnel: [w296 w297] -> w268
          tunnel: "Set Spike Position (in)" -> [w296 _]
          tunnel: [w296 w297] -> w266
          frame False {
          }
          frame True {
            w297 = 0.0
            n129 = property on="Set Spike Position (in)" class="Slide (strict)"("Value"=w297) -> ()  [unwired: 2 in, 2 out]
          }
        }
        "?" <- w266
        n130 = Build Array(w265) -> (w275:dbl[])
        n131 = Add(x="Set Spike Position (in)", y=-0.005) -> (x+y=w288:dbl)
        n132 = call <vilib>:"Interpolate 1D.vi"("xi"=w275, "X"=w274, "Y"=w273) -> ("yi"=w272:dbl[])  [unwired: 6 in, 2 out]
        n133 = Index Array(array=w272, index=0) -> (element=→"Output Mach #\n(For Reference Only)":dbl)
        n134 = Add(x="Set Spike Position (in)", y=0.005) -> (x+y=w290:dbl)
        n135 = In Range and Coerce(upper limit=w290, x=w265, lower limit=w288) -> (In Range?=w291:bool)  [unwired: 1 out]
        n136 = Subtract(x=w265, y=w268) -> (x-y=w292:dbl)
        "?" <- w292
        n137 = case shown="False" w291 {
          tunnel: w292 -> [w317 _]
          tunnel: w282 -> [w315 w338]
          tunnel: [w313 w335] -> w286
          tunnel: w281 -> [w316 w334]
          tunnel: [w314 w333] -> w285
          tunnel: [w310 w330] -> w284
          tunnel: w283 -> [w312 w337]
          frame False {
            n138 = call "Is Value Changed.vim"("value"=w312) -> ("changed or first call?"=w311:bool)
            n139 = Greater Than 0?(x=w317) -> (x > 0?=w318:bool)
            n140 = case shown="False" w318 {
              tunnel: [w324 w327] -> w310
              frame False {
                n141 = Concatenate Strings("CW" ("write buffer"), "\n" ("write buffer")) -> (w324:string)
              }
              frame True {
                n142 = Concatenate Strings("CCW" ("write buffer"), "\n" ("write buffer")) -> (w327:string)
              }
            }
            n143 = case shown="False" w311 {
              tunnel: w316 -> [_ w323]
              tunnel: w315 -> [_ w322]
              tunnel: [_ w321] -> w314
              tunnel: [_ w320] -> w313
              tunnel: w310 -> [_ w319]
              frame False {
              }
              frame True {
                n144 = VISA Write(VISA resource name=w322, write buffer=w319, error in (no error)=w323) -> (VISA resource name out=w320:refnum<visa-resource-name>, error out=w321:errorcluster)  [unwired: 1 out]
              }
            }
          }
          frame True {
            n145 = call "Is Value Changed.vim"("value"=w337) -> ("changed or first call?"=w336:bool)
            n146 = Concatenate Strings("STOP" ("write buffer"), "\n" ("write buffer")) -> (w330:string)
            n147 = case shown="True" w336 {
              tunnel: w330 -> [_ w343]
              tunnel: w338 -> [_ w342]
              tunnel: [_ w341] -> w335
              tunnel: w334 -> [_ w340]
              tunnel: [_ w339] -> w333
              frame False {
              }
              frame True {
                n148 = VISA Write(VISA resource name=w342, write buffer=w343, error in (no error)=w340) -> (VISA resource name out=w341:refnum<visa-resource-name>, error out=w339:errorcluster)  [unwired: 1 out]
              }
            }
          }
        }
        "Motor Signal" <- w283
      }
      frame "Set Mach # mode" {
        w365 = 1 items=["nearest", "linear", "spline", "cubic Hermite", "Lagrange"] ("method")
        n149 = case shown="\"Mach 3.0 Spike\"" w369 {
          tunnel: w355 -> [w416 _]
          tunnel: [w418 w423] -> w360
          tunnel: [w417 w424] -> w359
          tunnel: w356 -> [_ w420]
          frame "Mach 2.1 Spike", Default {
            n150 = Transpose 2D Array(2D array=w416) -> (transposed array=w415:dbl[][])
            n151 = Index Array(array=w415, index (row)=1) -> (element=w418:dbl[])  [unwired: 1 in]
            n152 = Index Array(array=w415, index (row)=0) -> (element=w417:dbl[])  [unwired: 1 in]
          }
          frame "Mach 3.0 Spike" {
            n153 = Transpose 2D Array(2D array=w420) -> (transposed array=w419:dbl[][])
            n154 = Index Array(array=w419, index (row)=1) -> (element=w423:dbl[])  [unwired: 1 in]
            n155 = Index Array(array=w419, index (row)=0) -> (element=w424:dbl[])  [unwired: 1 in]
          }
        }
        n156 = case shown="False" "?" {
          tunnel: w378 -> [w461 w469]
          tunnel: [w460 w468] -> w379
          tunnel: w376 -> [_ w464]
          tunnel: w377 -> [_ w463]
          frame False {
            n157 = Enqueue Element(queue=w461, element=T1."Set Mach # mode") -> (queue out=w460:refnum<queue>)  [unwired: 2 in, 2 out]
          }
          frame True {
            n158 = Concatenate Strings("STOP" ("write buffer"), "\n" ("write buffer")) -> (w467:string)
            n159 = VISA Write(VISA resource name=w464, write buffer=w467, error in (no error)=w463) -> ()  [unwired: 3 out]
            n160 = Enqueue Element(queue=w469, element=T1."Save Data") -> (queue out=w468:refnum<queue>)  [unwired: 2 in, 2 out]
          }
        }
        n161 = case shown="\"Mach 2.1 Spike\", Default" w369 {
          tunnel: "Select Mach Number" -> [w395 w410]
          tunnel: [w394 w407] -> w367
          tunnel: w356 -> [_ w406]
          tunnel: w355 -> [w390 _]
          frame "Mach 2.1 Spike", Default {
            w391 = 0.05 ("y")
            w389 = 0 ("index")
            n162 = Index Array(array=w395, index=w389) -> (element=w397:dbl)
            n163 = Index Array(array=w390, index (row)=w389) -> (element=w388:dbl[])  [unwired: 1 in]
            n164 = Array Max & Min(array=w388) -> (max value=w393:dbl, min value=w392:dbl)  [unwired: 2 out]
            n165 = Add(x=w393, y=w391) -> (x+y=w387:dbl)
            n166 = Subtract(x=w392, y=w391) -> (x-y=w386:dbl)
            n167 = In Range and Coerce(upper limit=w387, x=w397, lower limit=w386) -> (In Range?=w396:bool)  [unwired: 1 out]
            n168 = case shown="True" w396 {
              tunnel: w395 -> [_ w398]
              tunnel: [_ w398] -> w394
              frame False {
              }
              frame True {
              }
            }
          }
          frame "Mach 3.0 Spike" {
            w400 = 0.05 ("y")
            n169 = Index Array(array=w406, index (row)=0) -> (element=w404:dbl[])  [unwired: 1 in]
            n170 = Index Array(array=w410, index=0) -> (element=w409:dbl)
            n171 = Array Max & Min(array=w404) -> (max value=w403:dbl, min value=w401:dbl)  [unwired: 2 out]
            n172 = Add(x=w403, y=w400) -> (x+y=w402:dbl)
            n173 = Subtract(x=w401, y=w400) -> (x-y=w399:dbl)
            n174 = In Range and Coerce(upper limit=w402, x=w409, lower limit=w399) -> (In Range?=w408:bool)  [unwired: 1 out]
            n175 = case shown="False" w408 {
              tunnel: w410 -> [_ w412]
              tunnel: [_ w412] -> w407
              frame False {
              }
              frame True {
              }
            }
          }
        }
        n176 = Build Array(w358) -> (w357:dbl[])
        n177 = call <vilib>:"Interpolate 1D.vi"("xi"=w357, "X"=w360, "Y"=w359) -> ("yi"=w363:dbl[])  [unwired: 6 in, 2 out]
        n178 = Index Array(array=w363, index=0) -> (element=→"Output Mach #\n(For Reference Only)":dbl)
        n179 = call <vilib>:"Interpolate 1D.vi"("method"=w365, "xi"=w367, "X"=w359, "Y"=w360) -> ("yi"=w366:dbl[])  [unwired: 5 in, 2 out]
        n180 = Index Array(array=w366, index=0) -> (element=w364:dbl)
        n181 = Subtract(x=w358, y=w364) -> (x-y=w385:dbl)
        "?" <- w385
        n182 = Add(x=w364, y=0.005) -> (x+y=w383:dbl)
        n183 = Add(x=w364, y=-0.005) -> (x+y=w381:dbl)
        n184 = In Range and Coerce(upper limit=w383, x=w358, lower limit=w381) -> (In Range?=w384:bool)  [unwired: 1 out]
        n185 = case shown="False" w384 {
          tunnel: w385 -> [w432 _]
          tunnel: w376 -> [w430 w453]
          tunnel: [w428 w450] -> w375
          tunnel: w377 -> [w431 w449]
          tunnel: [w429 w448] -> w374
          tunnel: [w425 w445] -> w373
          tunnel: w372 -> [w427 w452]
          frame False {
            n186 = call "Is Value Changed.vim"("value"=w427) -> ("changed or first call?"=w426:bool)
            n187 = Greater Than 0?(x=w432) -> (x > 0?=w433:bool)
            n188 = case shown="True" w433 {
              tunnel: [w439 w442] -> w425
              frame False {
                n189 = Concatenate Strings("CW" ("write buffer"), "\n" ("write buffer")) -> (w439:string)
              }
              frame True {
                n190 = Concatenate Strings("CCW" ("write buffer"), "\n" ("write buffer")) -> (w442:string)
              }
            }
            n191 = case shown="False" w426 {
              tunnel: w431 -> [_ w438]
              tunnel: w430 -> [_ w437]
              tunnel: [_ w436] -> w429
              tunnel: [_ w435] -> w428
              tunnel: w425 -> [_ w434]
              frame False {
              }
              frame True {
                n192 = VISA Write(VISA resource name=w437, write buffer=w434, error in (no error)=w438) -> (VISA resource name out=w435:refnum<visa-resource-name>, error out=w436:errorcluster)  [unwired: 1 out]
              }
            }
          }
          frame True {
            n193 = call "Is Value Changed.vim"("value"=w452) -> ("changed or first call?"=w451:bool)
            n194 = Concatenate Strings("STOP" ("write buffer"), "\n" ("write buffer")) -> (w445:string)
            n195 = case shown="False" w451 {
              tunnel: w445 -> [_ w458]
              tunnel: w453 -> [_ w457]
              tunnel: [_ w456] -> w450
              tunnel: w449 -> [_ w455]
              tunnel: [_ w454] -> w448
              frame False {
              }
              frame True {
                n196 = VISA Write(VISA resource name=w457, write buffer=w458, error in (no error)=w455) -> (VISA resource name out=w456:refnum<visa-resource-name>, error out=w454:errorcluster)  [unwired: 1 out]
              }
            }
          }
        }
        "Motor Signal" <- w372
      }
      frame "Idle Mode" {
        n197 = event shown="[2] \"Flight Profile Mode\": Value Change" {
          selector: _ -> [_ _ _]
          dyn-events: _ -> [_ _ _]
          timeout: _ -> [_ _ _]
          tunnel: w481 -> [w484 w487 w490]
          tunnel: [w483 w486 w489] -> w480
          event "Manual Positioning Mode": Value Change {
            n198 = event-data() -> ()  [unwired: 1 in, 6 out]
            n199 = Enqueue Element(queue=w484, element=T1."Manual Positioning Mode") -> (queue out=w483:refnum<queue>)  [unwired: 2 in, 2 out]
          }
          event "Set Mach # Mode": Value Change {
            n200 = event-data() -> ()  [unwired: 1 in, 6 out]
            n201 = Enqueue Element(queue=w487, element=T1."Set Mach # mode") -> (queue out=w486:refnum<queue>)  [unwired: 2 in, 2 out]
          }
          event "Flight Profile Mode": Value Change {
            n202 = event-data() -> ()  [unwired: 1 in, 6 out]
            n203 = Enqueue Element(queue=w490, element=T1."Flight Profile Mode") -> (queue out=w489:refnum<queue>)  [unwired: 2 in, 2 out]
          }
        }
        n204 = property on="Loop Iteration" class="DigNum (strict)"("Value"=0 ("Loop Iteration 2")) -> ()  [unwired: 2 in, 2 out]
        n205 = Concatenate Strings("STOP" ("write buffer"), "\n" ("write buffer")) -> (w475:string)
        n206 = property class="Bool"("DisabledEnum"=T3."Disabled" ("Disabled")) -> ()  [unwired: 2 in, 2 out]
        n207 = property on="Manual Positioning Mode" class="Bool"("DisabledEnum"=T3."Enabled" ("Disabled")) -> ()  [unwired: 2 in, 2 out]
        n208 = property on="Set Mach # Mode" class="Bool"("DisabledEnum"=T3."Enabled" ("Disabled")) -> ()  [unwired: 2 in, 2 out]
        n209 = property class="Bool"("DisabledEnum"=T3."Disabled" ("Disabled")) -> ()  [unwired: 2 in, 2 out]
        n210 = VISA Write(VISA resource name=w472, write buffer=w475, error in (no error)=w471) -> ()  [unwired: 3 out]
      }
      frame "Flight Profile Mode" {
        w552 = 1 items=["nearest", "linear", "spline", "cubic Hermite", "Lagrange"] ("method")
        n211 = case shown="\"Mach 2.1 Spike\", Default" w550 {
          tunnel: w517 -> [w647 _]
          tunnel: [w649 w654] -> w535
          tunnel: [w648 w655] -> w534
          tunnel: w518 -> [_ w651]
          frame "Mach 2.1 Spike", Default {
            n212 = Transpose 2D Array(2D array=w647) -> (transposed array=w646:dbl[][])
            n213 = Index Array(array=w646, index (row)=1) -> (element=w649:dbl[])  [unwired: 1 in]
            n214 = Index Array(array=w646, index (row)=0) -> (element=w648:dbl[])  [unwired: 1 in]
          }
          frame "Mach 3.0 Spike" {
            n215 = Transpose 2D Array(2D array=w651) -> (transposed array=w650:dbl[][])
            n216 = Index Array(array=w650, index (row)=1) -> (element=w654:dbl[])  [unwired: 1 in]
            n217 = Index Array(array=w650, index (row)=0) -> (element=w655:dbl[])  [unwired: 1 in]
          }
        }
        n218 = Equal To 0?(x=w505) -> (x = 0?=w504:bool)
        n219 = case shown="True" "?" {
          tunnel: w564 -> [w658 w666]
          tunnel: [w657 w665] -> w513
          tunnel: w546 -> [_ w661]
          tunnel: w545 -> [_ w660]
          frame False {
            n220 = Enqueue Element(queue=w658, element=T1."Flight Profile Mode") -> (queue out=w657:refnum<queue>)  [unwired: 2 in, 2 out]
          }
          frame True {
            n221 = Concatenate Strings("STOP" ("write buffer"), "\n" ("write buffer")) -> (w664:string)
            n222 = VISA Write(VISA resource name=w661, write buffer=w664, error in (no error)=w660) -> ()  [unwired: 3 out]
            n223 = Enqueue Element(queue=w666, element=T1."Save Data") -> (queue out=w665:refnum<queue>)  [unwired: 2 in, 2 out]
          }
        }
        n224 = case shown="True" w504 {
          tunnel: w505 -> [w569 _]
          tunnel: [w568 _] -> w515
          frame False {
            n225 = call "Is Value Changed.vim"("value"=w569) -> ("changed or first call?"=w568:bool)
          }
          frame True {
          }
        }
        n226 = Transpose 2D Array(2D array="?") -> (transposed array=w508:dbl[][])
        n227 = property class="Bool"("DisabledEnum"=T3."Enabled" ("Disabled")) -> ()  [unwired: 2 in, 2 out]
        n228 = property on="Set Mach # Mode" class="Bool"("DisabledEnum"=T3."Disabled" ("Disabled")) -> ()  [unwired: 2 in, 2 out]
        n229 = Index Array(array=w508, index (row)=0) -> (element=w524:dbl[])  [unwired: 1 in]
        n230 = Index Array(array=w508, index (row)=1) -> (element=w526:dbl[])  [unwired: 1 in]
        n231 = Index Array(array=w526, index="Loop Iteration") -> (element=w525:dbl)
        n232 = Index Array(array=w524, index="Loop Iteration") -> (element=w512:dbl)
        n233 = Build Array(w499) -> (w536:dbl[])
        n234 = call <vilib>:"Interpolate 1D.vi"("xi"=w536, "X"=w535, "Y"=w534) -> ("yi"=w533:dbl[])  [unwired: 6 in, 2 out]
        n235 = Build Array(w512) -> (w523:dbl[])
        n236 = First Call?() -> (First Call?: T/F=w537:bool)
        n237 = case shown="\"Mach 2.1 Spike\", Default" w550 {
          tunnel: w523 -> [w627 w642]
          tunnel: [w626 w639] -> w554
          tunnel: w518 -> [_ w634]
          tunnel: w517 -> [w619 _]
          frame "Mach 2.1 Spike", Default {
            w623 = 0.05 ("y")
            w618 = 0 ("index")
            n238 = Index Array(array=w627, index=w618) -> (element=w629:dbl)
            n239 = Index Array(array=w619, index (row)=w618) -> (element=w622:dbl[])  [unwired: 1 in]
            n240 = Array Max & Min(array=w622) -> (max value=w625:dbl, min value=w624:dbl)  [unwired: 2 out]
            n241 = Add(x=w625, y=w623) -> (x+y=w621:dbl)
            n242 = Subtract(x=w624, y=w623) -> (x-y=w620:dbl)
            n243 = In Range and Coerce(upper limit=w621, x=w629, lower limit=w620) -> (In Range?=w628:bool)  [unwired: 1 out]
            n244 = case shown="True" w628 {
              tunnel: w627 -> [_ w630]
              tunnel: [_ w630] -> w626
              frame False {
              }
              frame True {
              }
            }
          }
          frame "Mach 3.0 Spike" {
            w636 = 0.05 ("y")
            w631 = 0 ("index")
            n245 = Index Array(array=w642, index=w631) -> (element=w641:dbl)
            n246 = Index Array(array=w634, index (row)=w631) -> (element=w635:dbl[])  [unwired: 1 in]
            n247 = Array Max & Min(array=w635) -> (max value=w638:dbl, min value=w637:dbl)  [unwired: 2 out]
            n248 = Add(x=w638, y=w636) -> (x+y=w633:dbl)
            n249 = Subtract(x=w637, y=w636) -> (x-y=w632:dbl)
            n250 = In Range and Coerce(upper limit=w633, x=w641, lower limit=w632) -> (In Range?=w640:bool)  [unwired: 1 out]
            n251 = case shown="True" w640 {
              tunnel: w642 -> [_ w643]
              tunnel: [_ w643] -> w639
              frame False {
              }
              frame True {
              }
            }
          }
        }
        n252 = case shown="False" w537 {
          tunnel: [w581 _] -> w528
          tunnel: w538 -> [w581 _]
          tunnel: [w580 _] -> w519
          tunnel: w515 -> [w580 _]
          frame False {
          }
          frame True {
          }
        }
        n253 = Equal To 0?(x=w512) -> (x = 0?=w511:bool)
        n254 = Index Array(array=w533, index=0) -> (element=w500:dbl)
        "?" <- w500
        n255 = case shown="True" w511 {
          tunnel: [w570 w572] -> w514
          tunnel: w513 -> [w570 w574]
          frame False {
          }
          frame True {
            n256 = Dequeue Element(queue=w574) -> (queue out=w573:refnum<queue>)  [unwired: 2 in, 3 out]
            n257 = Enqueue Element(queue=w573, element=T1."Save Data") -> (queue out=w572:refnum<queue>)  [unwired: 2 in, 2 out]
          }
        }
        n258 = Insert Into Array(array=w507, new element=w500) -> (w506:dbl[])  [unwired: 1 in]
        n259 = Build Array(w500) -> (w503:dbl[])
        n260 = Build Array(w500, w499) -> (w495:dbl[])
        n261 = Concatenate Strings("STOP" ("string"), "\n" ("string")) -> (w529:string)
        n262 = Equal?(x=w528, y=w529) -> (x = y?=w527:bool)
        n263 = case shown="False" w519 {
          frame False {
          }
          frame True {
            n264 = property on="Loop Iteration" class="DigNum (strict)"() -> ("Value"=w578:i32)  [unwired: 2 in, 2 out]
            n265 = Add(x=1, y=w578) -> (x+y=w576:i32)
            n266 = property on="Loop Iteration" class="DigNum (strict)"("Value"=w576) -> ()  [unwired: 2 in, 2 out]
          }
        }
        n267 = Insert Into Array(array=w501, new element=w503) -> (w502:dbl[])  [unwired: 1 in]
        "Waveform Chart" <- w502
        n268 = Array Size(array=w495) -> (size(s)=w494:i32)
        n269 = case shown="False" w527 {
          tunnel: [_ w579] -> w516
          tunnel: w525 -> [_ w579]
          frame False {
          }
          frame True {
          }
        }
        n270 = for {
          N: w494 -> [_]
          tunnel: w495 -> [w567] mode=indexing
          tunnel: [w565] -> w498 mode=indexing
          n271 = Number To Decimal String(number=w567, width (-)=i16 5) -> (decimal integer string=w565:string)
        }
        n272 = Format Date/Time String(time format string (%c)="%H%M%S%3u") -> (date/time string=w491:string)  [unwired: 2 in]
        n273 = case shown="False" w515 {
          tunnel: [w575 _] -> w510
          tunnel: w516 -> [w575 _]
          frame False {
          }
          frame True {
          }
        }
        "Mach # duration (s)" <- w510
        n274 = Insert Into Array(array=w498, new element=w491) -> (w493:string[])  [unwired: 1 in]
        n275 = Build Array (concatenate)(w493, w496) -> (w497:string[][])
        n276 = Multiply(x=1000.0, y=w510) -> (x*y=w522:dbl)
        n277 = call <vilib>:"Interpolate 1D.vi"("method"=w552, "xi"=w554, "X"=w534, "Y"=w535) -> ("yi"=w553:dbl[])  [unwired: 5 in, 2 out]
        n278 = Wait (ms)(milliseconds to wait=w522) -> ()  [unwired: 1 out]
        n279 = Index Array(array=w553, index=0) -> (element=w551:dbl)
        n280 = Subtract(x=w499, y=w551) -> (x-y=→"?":dbl)
        n281 = Add(x=w551, y=0.005) -> (x+y=w559:dbl)
        n282 = Add(x=w551, y=-0.005) -> (x+y=w557:dbl)
        n283 = In Range and Coerce(upper limit=w559, x=w499, lower limit=w557) -> (In Range?=w547:bool)  [unwired: 1 out]
        n284 = case shown="False" w547 {
          tunnel: w499 -> [w591 _]
          tunnel: w546 -> [w589 w612]
          tunnel: [w587 w609] -> w549
          tunnel: w545 -> [w590 w608]
          tunnel: [w588 w607] -> w548
          tunnel: [w584 w604] -> w543
          tunnel: w538 -> [w586 w611]
          frame False {
            n285 = call "Is Value Changed.vim"("value"=w586) -> ("changed or first call?"=w585:bool)
            n286 = Greater Than 0?(x=w591) -> (x > 0?=w592:bool)
            n287 = case shown="True" w592 {
              tunnel: [w598 w601] -> w584
              frame False {
                n288 = Concatenate Strings("CW" ("write buffer"), "\n" ("write buffer")) -> (w598:string)
              }
              frame True {
                n289 = Concatenate Strings("CCW" ("write buffer"), "\n" ("write buffer")) -> (w601:string)
              }
            }
            n290 = case shown="False" w585 {
              tunnel: w590 -> [_ w597]
              tunnel: w589 -> [_ w596]
              tunnel: [_ w595] -> w588
              tunnel: [_ w594] -> w587
              tunnel: w584 -> [_ w593]
              frame False {
              }
              frame True {
                n291 = VISA Write(VISA resource name=w596, write buffer=w593, error in (no error)=w597) -> (VISA resource name out=w594:refnum<visa-resource-name>, error out=w595:errorcluster)  [unwired: 1 out]
              }
            }
          }
          frame True {
            n292 = call "Is Value Changed.vim"("value"=w611) -> ("changed or first call?"=w610:bool)
            n293 = Concatenate Strings("STOP" ("write buffer"), "\n" ("write buffer")) -> (w604:string)
            n294 = case shown="True" w610 {
              tunnel: w604 -> [_ w617]
              tunnel: w612 -> [_ w616]
              tunnel: [_ w615] -> w609
              tunnel: w608 -> [_ w614]
              tunnel: [_ w613] -> w607
              frame False {
              }
              frame True {
                n295 = VISA Write(VISA resource name=w616, write buffer=w617, error in (no error)=w614) -> (VISA resource name out=w615:refnum<visa-resource-name>, error out=w613:errorcluster)  [unwired: 1 out]
              }
            }
          }
        }
        n296 = Equal?(x=w543, y="STOP" ("write buffer")) -> (x = y?=w541:bool)
        n297 = case shown="False" w541 {
          tunnel: [w582 w583] -> w542
          tunnel: w543 -> [w582 w583]
          frame False {
          }
          frame True {
          }
        }
        "Motor Signal" <- w538
      }
      frame "Save Data" {
        n298 = Enqueue Element(queue=w679, element=T1."Idle Mode") -> (queue out=w677:refnum<queue>)  [unwired: 2 in, 2 out]
        n299 = call <vilib>:"Create Report.vi"("Report Type"=Report_Type."Excel" ("report type")) -> ("report out"=w676:refnum<class "NI_report.lvclass">)  [unwired: 13 in, 1 out]
        n300 = call <vilib>:"Three Button Dialog.vi"("Window Title (\"\")"="Save Control Values" ("Window Title (\"\")"), "Right Button Text (\"Cancel\")"="Mach Profile" ("Right Button Text (\"Cancel\")"), "Center Button Text (\"No\")"="Set Mach" ("Center Button Text (\"No\")"), "Left Button Text (\"Yes\")"="Manual" ("Left Button Text (\"Yes\")"), "message"="Save Data For Test Mode?") -> ("Which Button?"=w672:T5)  [unwired: 6 in]
        n301 = case shown="\"Left Button\", Default" w672 {
          tunnel: w676 -> [w681 w685 w686]
          tunnel: string[] ["Mach #", "Spike Position (in)", "Time (s)", ""] ("column headers") -> [w680 w683 w688]
          tunnel: w673 -> [w682 w684 w687]
          frame "Left Button", Default {
            n302 = call-poly <vilib>:"Excel Easy Table.vi"("report in"=w681, "text data"=w682, "column headers"=w680) -> ()  [unwired: 8 in, 5 out]
          }
          frame "Center Button" {
            n303 = call-poly <vilib>:"Excel Easy Table.vi"("report in"=w685, "text data"=w684, "column headers"=w683) -> ()  [unwired: 8 in, 5 out]
          }
          frame "Right Button" {
            n304 = call-poly <vilib>:"Excel Easy Table.vi"("report in"=w686, "text data"=w687, "column headers"=w688) -> ()  [unwired: 8 in, 5 out]
          }
        }
      }
    }
    "Set Motor RPM" <- "?"
  }
  n305 = Release Queue(queue=w21) -> ()  [unwired: 2 in, 3 out]
  n306 = call "LJM_Close.vi"("error in"=w29, "Handle"=w28) -> ("error out"=→"Labjack error":errorcluster)  [unwired: 9 in]
  n307 = Release Queue(queue=w20) -> ()  [unwired: 2 in, 3 out]
  n308 = VISA Close(VISA resource name=w11, error in (no error)=w10) -> (error out=→"Arduino Error":errorcluster)
